vi "UDPConnect.vi"(4 "data":string, 5 "Optitrack Parameters":T1={"Optitrack IP"="130.207.141.229", "Optitrack Port"=1520, "timeout (sec)"=80}, 6 "error in (no error)":errorcluster, 8 "Action":enum16{"open port", "close port", "send data"}(ring)=enum."send data", 9 "connection ID":refnum<k16>) -> (0 "error out":errorcluster, 3 "connection ID out":refnum<k16>)   [LabVIEW 2012]
panel:
  # "v"
  # "130.207.141.229"
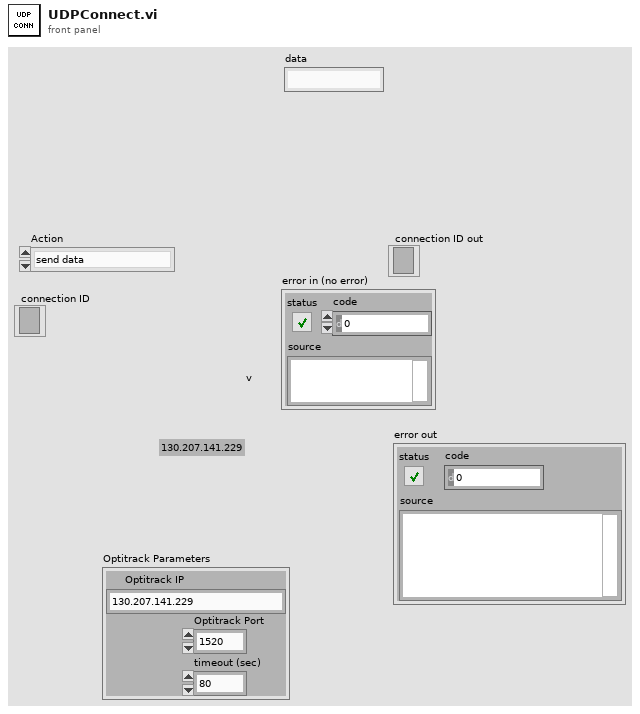
[diagram p1: front panel]
types:
  T1 = cluster{"Optitrack IP":string, "Optitrack Port":u16, "timeout (sec)":u32}
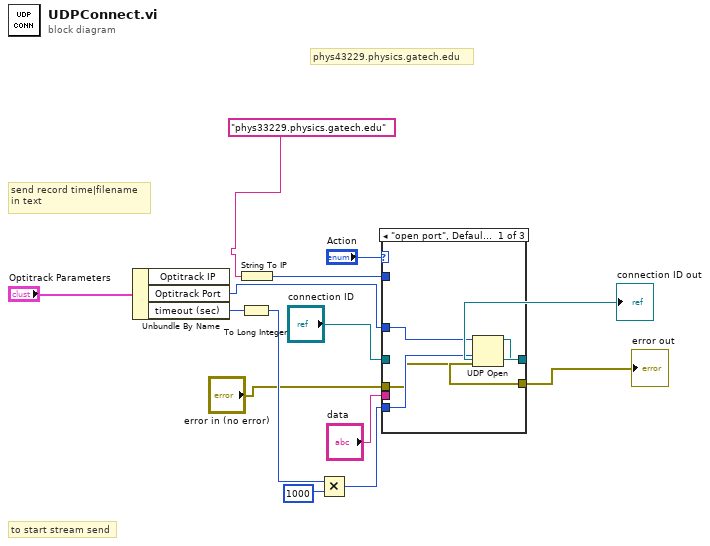
[diagram p0: block diagram]
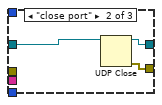
[diagram p2: hidden frame]
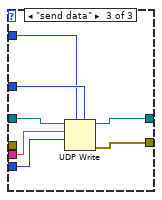
[diagram p3: hidden frame]
diagram:
  # "phys43229.physics.gatech.edu"
  # "send record time|filename\nin text"
  # "to start stream send"
  n1 = Unbundle By Name("Optitrack Parameters") -> ("Optitrack Port"=w8:u16, "timeout (sec)"=w5:u32)  [unwired: 1 out]
  n2 = To Long Integer(number=w5) -> (32bit integer=w4:i32)
  n3 = String To IP(1:"phys33229.physics.gatech.edu" ("data")) -> (0:w7:u32)
  n4 = Multiply(x=w4, y=1000) -> (x*y=w3:i32)
  n5 = case shown="\"open port\", Default" "Action" {
    tunnel: "connection ID" -> [_ w22 w29]
    tunnel: [w17 w21 w25] -> w11
    tunnel: [w18 w20 w26] -> w10
    tunnel: "data" -> [_ _ w28]
    tunnel: w7 -> [_ _ w23]
    tunnel: w8 -> [w19 _ w24]
    tunnel: w3 -> [w16 _ w27]
    tunnel: "error in (no error)" -> [w15 _ _]
    frame "open port", Default {
      n6 = UDP Open(8:w15, 9:w16, 11:w19) -> (port=w18:refnum<k16>, 0:w17:errorcluster)  [unwired: 2 in, 1 out]
    }
    frame "close port" {
      n7 = UDP Close(connection ID=w22) -> (connection ID out=w20:refnum<k16>, error out=w21:errorcluster)  [unwired: 1 in]
    }
    frame "send data" {
      n8 = UDP Write(address=w23, port or service name=w24, connection ID=w29, data in=w28, 9:w27) -> (error out=w25:errorcluster, 3:w26:refnum<k16>)  [unwired: 1 in]
    }
  }
  "error out" <- w11
  "connection ID out" <- w10
